vi "FindFirstTag with Attributes.vi"(6 "max offset":i32, 8 "offset (0)":i32, 11 "XML String In":string) -> (0 "offset past match":i32, 2 "start tag":T1, 4 "case":enum16{"Start Tag", "Empty Element", "Content"}(ring), 5 "element name":string, 7 "Attributes":cluster{"Keys":string[], "Values":string[]})   [LabVIEW 2011]
doc: "This VI finds the first XML tag (start tag or empty element tag) in the string and returns:\n\nbefore tag - portion of string prior to the tag\ntag - the contents of the tag including angle brackets (<,>)\nafter tag - portion of string found after the end of the tag\noffset past match - index in string of the first character of after substring\nelement name - the name (including namespace if applicable) of the element\ncase - whether a \"Start Tag\", \"Empty Element\", or \"Content\" (no tags) was found"
uses:
  Type Defs/Node Info - Cluster.ctl
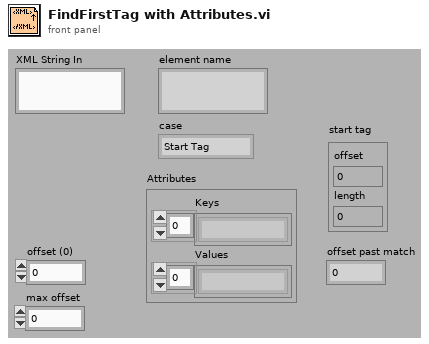
[diagram p1: front panel]
types:
  T1 = typedef "Node Info - Cluster.ctl" = cluster{"offset":i32, "length":i32}
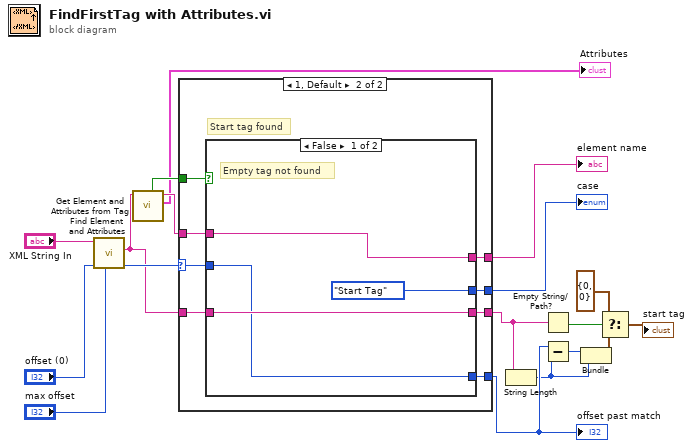
[diagram p0: block diagram]
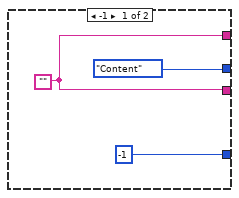
[diagram p2: hidden frame]
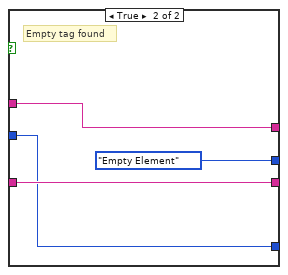
[diagram p3: hidden frame]
diagram:
  n1 = call "Find Element and Attributes.vi"("max offset"="max offset", "offset (0)"="offset (0)", "XML String In"="XML String In") -> ("offset past match"=w18:i32, "tag with attributes"=w13:string)  [unwired: 7 in]
  n2 = call "Get Element and Attributes from Tag.vi"("tag with attributes"=w13) -> ("Attributes"=→"Attributes":cluster{"Keys":string[], "Values":string[]}, "element name"=w12:string, "empty element?"=w11:bool)  [unwired: 7 in, 1 out]
  n3 = case shown="1, Default" w18 {
    selector: w18 -> [_ w28]
    tunnel: [enum16{"Start Tag", "Empty Element", "Content"}."Content" w29] -> w14
    tunnel: w13 -> [_ w27]
    tunnel: [w20 w26] -> w8
    tunnel: w12 -> [_ w25]
    tunnel: [w20 w24] -> w16
    tunnel: [-1 ("offset past match") w23] -> w7
    tunnel: w11 -> [_ w22]
    frame -1 {
      w20 = ""
    }
    frame 1, Default {
      # "Start tag found"
      n4 = case shown="False" w22 {
        tunnel: [enum16{"Start Tag", "Empty Element", "Content"}."Start Tag" enum16{"Start Tag", "Empty Element", "Content"}."Empty Element"] -> w29
        tunnel: w28 -> [w31 w34]
        tunnel: w27 -> [w33 w36]
        tunnel: [w33 w36] -> w26
        tunnel: w25 -> [w32 w35]
        tunnel: [w32 w35] -> w24
        tunnel: [w31 w34] -> w23
        frame False {
          # "Empty tag not found"
        }
        frame True {
          # "Empty tag found"
        }
      }
    }
  }
  "element name" <- w16
  "offset past match" <- w7
  "case" <- w14
  n5 = String Length(string=w8) -> (length=w5:i32)
  n6 = Empty String/Path?(string/path=w8) -> (empty?=w9:bool)
  n7 = Subtract(x=w7, y=w5) -> (x-y=w6:i32)
  n8 = Bundle(w6, w5) -> (w4:cluster{i32, i32})  [unwired: 1 in]
  n9 = Select(t=cluster{i32, i32} {0, 0}, s=w9, f=w4) -> (s? t:f=→"start tag":cluster{i32, i32})
